vi "DistanceCount.vi"() -> ()   [LabVIEW 2018]
panel:
  in  "distanceCount":dbl
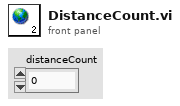
[diagram p1: front panel]
diagram:
